vi "ALLPROP1_Test.vi"(8 "error in (no error)":errorcluster) -> (0 "error out":errorcluster, 3 "Passed?":bool)   [LabVIEW 2021]
panel:
  out "Inputs":T1
  in  "Fluid of interest":string="HELIUM.FLD"
  out "Outputs":cluster{"C":dbl[], "ierr":i32, "herr":string}={"C"=[], "ierr"=0, "herr"="                                                                                                                                                                                                                                                               "}
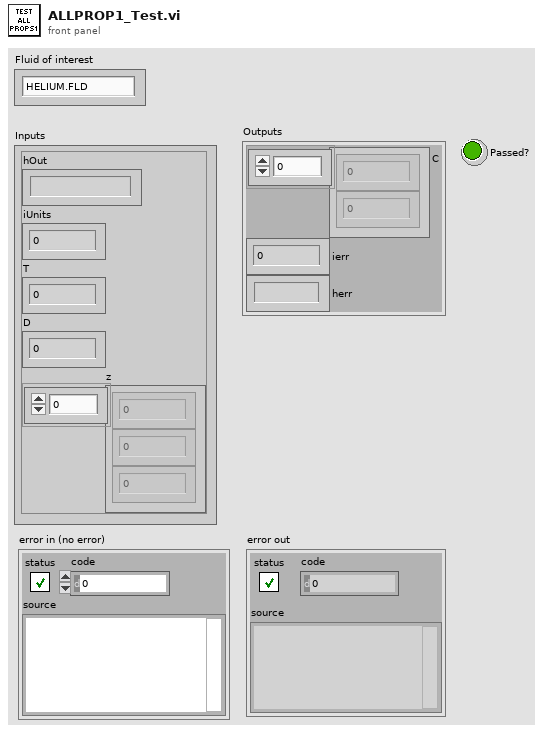
[diagram p1: front panel]
types:
  T1 = cluster{"hOut":string, "iUnits":i32, "T":dbl, "D":dbl, "z":dbl[]}
  T2 = typedef "Mixture Composition cluster_d.ctl" = cluster{"Mixture Name":string, "Molecular weight (g/mol)":dbl, "Critical temperature (K)":dbl, "Critical Pressure (kPa)":dbl, "Critical Density (mol/L)":dbl, "# Components":i32, "Fluid File Paths":path[], "Component molar fractions":dbl[], "Refprop Main Directory":path, "DLL Version Number":dbl}
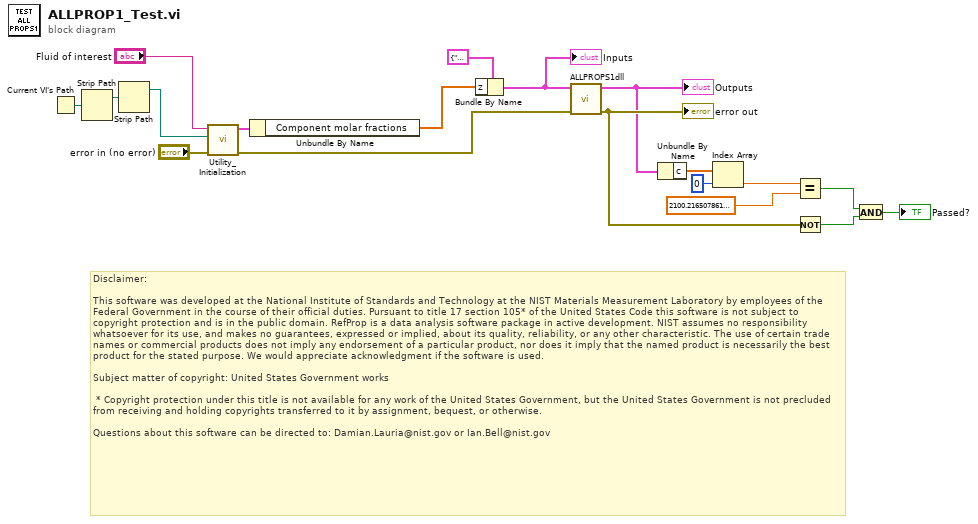
[diagram p0: block diagram]
diagram:
  # "Disclaimer:\n\nThis software was developed at the National Institute of Standards and Technology at the NIST Materials Measurement Laboratory by employees of the Federal Government in the course of their official duties. Pursuant to title 17 section 105* of the United States Code this software is not subject to copyright protection and is in the public domain. RefProp is a data analysis software package in active development. NIST assumes no responsibility whatsoever for its use, and makes no guarantees, expressed or implied, about its quality, reliability, or any other characteristic. The use of certain trade names or commercial products does not imply any endorsement of a particular product, nor does it imply that the named product is necessarily the best product for the stated purpose. We would appreciate acknowledgment if the software is used.\n \nSubject matter of copyright: United States Government works\n  \n * Copyright protection under this title is not available for any work of the United States Government, but the United States Government is not precluded from receiving and holding copyrights transferred to it by assignment, bequest, or otherwise.\n\nQuestions about this software can be directed to: Damian.Lauria@nist.gov or Ian.Bell@nist.gov"
  n1 = Current VI's Path() -> (path=w5:path)
  n2 = Strip Path(path=w5) -> (stripped path=w4:path)  [unwired: 1 out]
  n3 = Strip Path(path=w4) -> (stripped path=w3:path)  [unwired: 1 out]
  n4 = call "Utility_Initialization.vi"("error in (no error)"="error in (no error)", "path"=w3, "Fluidofinterest"="Fluid of interest") -> ("error out"=w17:errorcluster, "Mixure Cluster out"=w2:T2)  [unwired: 6 in, 1 out]
  n5 = Unbundle By Name(w2) -> ("Component molar fractions"=w7:dbl[])
  n6 = Bundle By Name(cluster=T1 {"hOut"="H", "iUnits"=0, "T"=100.0, "D"=0.179, "z"=[0.697616, 0.302385]} ("Inputs"), "z"=w7) -> (w19:T1)
  "Inputs" <- w19
  n7 = call "ALLPROPS1dll.vi"("error in (no error)"=w17, "Inputs"=w19) -> ("error out"=w16:errorcluster, "Outputs"=w15:cluster{"c":dbl[], "ierr":i32, "herr":string})  [unwired: 8 in]
  "error out" <- w16
  "Outputs" <- w15
  n8 = Unbundle By Name(w15) -> ("c"=w13:dbl[])
  n9 = Index Array(array=w13, index=0) -> (element=w12:dbl)
  n10 = Equal?(x=w12, y=2100.216507861462 ("element")) -> (x = y?=w10:bool)
  n11 = Not(x=w16) -> (.not. x?=w11:bool)
  n12 = And(x=w10, y=w11) -> (x .and. y?=→"Passed?":bool)
